vi "VerStringTrim.vi"(1 "读取缓冲区":string) -> (0 "结果":string)   [LabVIEW 2013]
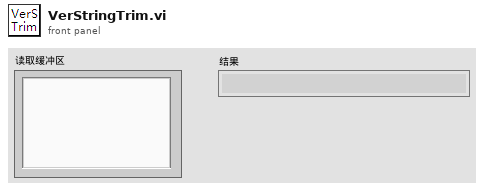
[diagram p1: front panel]
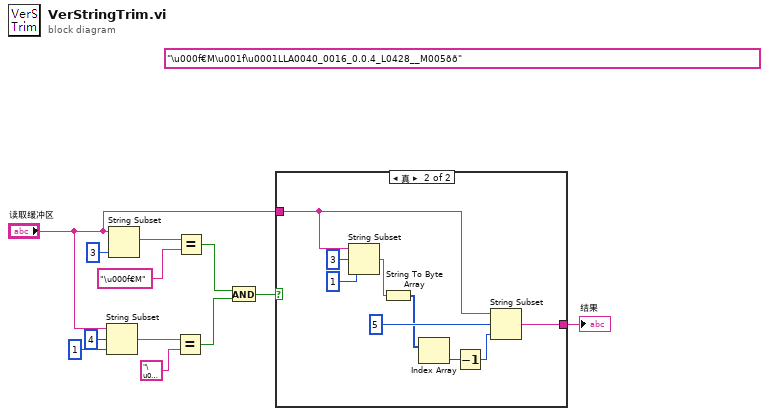
[diagram p0: block diagram]
diagram:
  (unwired) "\u000f€M\u001f\u0001LLA0040_0016_0.0.4_L0428__M005õð" ("读取缓冲区 2")
  n1 = String Subset(string="读取缓冲区", offset (0)=4 ("偏移量(0)"), length (rest)=1 ("长度（剩余）")) -> (substring=w7:string)
  n2 = String Subset(string="读取缓冲区", length (rest)=3 ("长度（剩余）")) -> (substring=w11:string)  [unwired: 1 in]
  n3 = Equal?(x=w7, y="\u0001") -> (x = y?=w4:bool)
  n4 = Equal?(x=w11, y="\u000f€M") -> (x = y?=w5:bool)
  n5 = And(x=w5, y=w4) -> (x .and. y?=w3:bool)
  n6 = case shown="真" w3 {
    tunnel: "读取缓冲区" -> [_ w19]
    tunnel: [_ w17] -> w1
    frame False {
    }
    frame True {
      n7 = String Subset(string=w19, offset (0)=3 ("偏移量(0)"), length (rest)=1 ("长度（剩余）")) -> (substring=w16:string)
      n8 = String To Byte Array(string=w16) -> (unsigned byte array=w15:u8[])
      n9 = Index Array(array=w15) -> (element=w14:u8)  [unwired: 1 in]
      n10 = Decrement(x=w14) -> (x-1=w13:u8)
      n11 = String Subset(string=w19, offset (0)=5 ("偏移量(0)"), length (rest)=w13) -> (substring=w17:string)
    }
  }
  "结果" <- w1
